vi "ex_AddColToHdngs.vi"(5 "new heading":string, 7 "headings":string[][](table)) -> (3 "headings out":string[][](table))   [LabVIEW 2017]
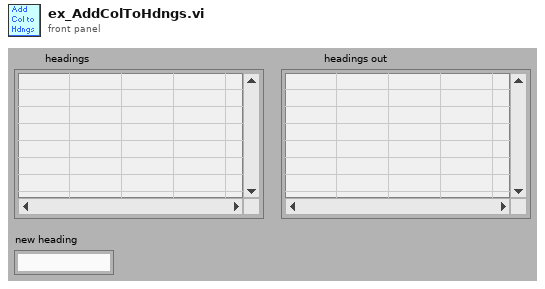
[diagram p1: front panel]
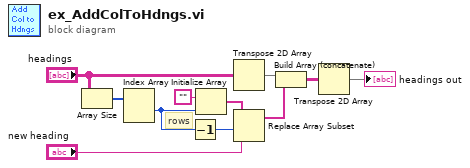
[diagram p0: block diagram]
diagram:
  # "rows"
  n1 = Array Size(array="headings") -> (size(s)=w11:i32[])
  n2 = Index Array(array=w11) -> (element #1=w9:i32)  [unwired: 2 in, 1 out]
  n3 = Decrement(x=w9) -> (x-1=w6:i32)
  n4 = Initialize Array("", w9) -> (w7:string[])
  n5 = Transpose 2D Array(2D array="headings") -> (transposed array=w2:string[][])
  n6 = Replace Array Subset(array=w7, new element="new heading", index=w6) -> (w4:string[])
  n7 = Build Array (concatenate)(w2, w4) -> (w3:string[][])
  n8 = Transpose 2D Array(2D array=w3) -> (transposed array=→"headings out":string[][])
